vi "onOffEx.vi"() -> ()   [LabVIEW 2017]
uses:
  <instrlib>/BK Precision XLN Series/BK Precision XLN Series.lvlib
panel:
  in  "Voltage Level (5.0 V)":dbl=5.0 format="%.3g"
  out "error out":errorcluster
  in  "VISA resource name":refnum<visa-resource-name>
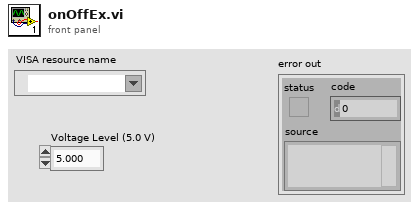
[diagram p1: front panel]
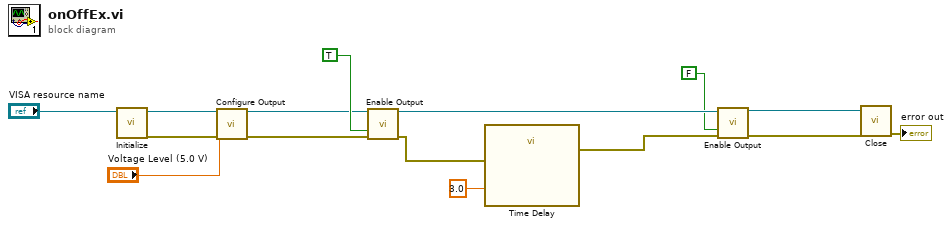
[diagram p0: block diagram]
diagram:
  n1 = call <instrlib>:"Initialize.vi"("VISA resource name"="VISA resource name") -> ("error out"=w3:errorcluster, "VISA resource name out"=w4:refnum<visa-resource-name>)  [unwired: 9 in]
  n2 = call <instrlib>:"Configure Output.vi"("VISA resource name"=w4, "Voltage Level (5.0 V)"="Voltage Level (5.0 V)", "error in (no error)"=w3) -> ("VISA resource name out"=w2:refnum<visa-resource-name>, "error out"=w1:errorcluster)  [unwired: 11 in]
  n3 = call <instrlib>:"Enable Output.vi"("VISA resource name"=w2, "Enable Output (F: False)"=TRUE, "error in (no error)"=w1) -> ("VISA resource name out"=w14:refnum<visa-resource-name>, "error out"=w8:errorcluster)  [unwired: 11 in]
  n4 = call "Time Delay"("error in (no error)"=w8, "Delay Time (s)"=3.0) -> ("error out"=w7:errorcluster)  [unwired: 9 in]
  n5 = call <instrlib>:"Enable Output.vi"("VISA resource name"=w14, "Enable Output (F: False)"=FALSE, "error in (no error)"=w7) -> ("VISA resource name out"=w13:refnum<visa-resource-name>, "error out"=w12:errorcluster)  [unwired: 11 in]
  n6 = call <instrlib>:"Close.vi"("error in (no error)"=w12, "VISA resource name"=w13) -> ("error out"=→"error out":errorcluster)  [unwired: 9 in]
